vi "Insert Step at Index.vi"(8 "error in (no error)":errorcluster, 9 "Index":i32, 10 "Step":refnum<class "Base Step.lvclass">, 11 "Sequence in":refnum<class "Sequence.lvclass">) -> (0 "error out":errorcluster, 3 "Sequence out":refnum<class "Sequence.lvclass">)   [LabVIEW 2024, in "Ramses Sequencer.lvlib" / "Sequence.lvclass"]
uses:
  Sequence.lvclass
  Base Step/Base Step.lvclass
  Sequence.lvclass/Sequence.ctl
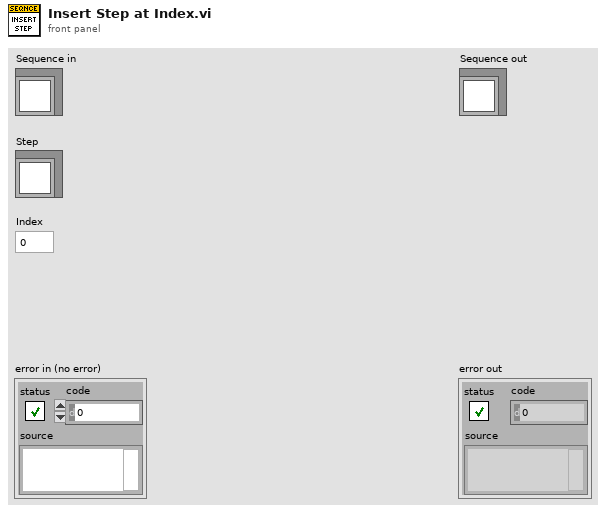
[diagram p1: front panel]
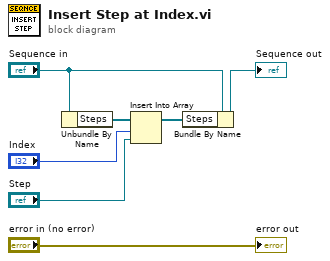
[diagram p0: block diagram]
diagram:
  n1 = Unbundle By Name("Sequence in") -> ("Steps"=w4:refnum<class "Base Step.lvclass">[])
  n2 = Insert Into Array(array=w4, index="Index", new element="Step") -> (w1:refnum<class "Base Step.lvclass">[])
  n3 = Bundle By Name(cluster="Sequence in", "Steps"=w1) -> (→"Sequence out":refnum<class "Sequence.lvclass">)
  "error out" <- "error in (no error)"
